vi "LaunchServerUI.vi"   [LabVIEW 2018, in "ServerUI.lvlib"]
uses:
  ServerUI.lvlib
  ServerUI/ServerUI.lvclass
  C:/Repos/AF_TCP_Example/TCP_Client/TCP_Client/TCP_Client.lvclass
  ClientUI/ClientUI/ClientUI.lvclass
  TCP_Client/TCP_Client/TCP_Client.lvclass
  C:/Program Files/National Instruments/LabVIEW 2018/vi.lib/ActorFramework/Actor/Actor.lvclass
  <vilib>/ActorFramework/Actor/Actor.lvclass
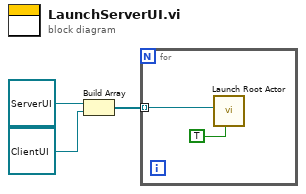
[diagram p0: block diagram]
diagram:
  n1 = Build Array(refnum<class "ServerUI.lvclass"> refnum ("ServerUI.lvlib:ServerUI.lvclass"), refnum<class "ClientUI.lvclass"> refnum ("ClientUI.lvlib:ClientUI.lvclass")) -> (w2:refnum<class "TCP_Client.lvclass">[])
  n2 = for {
    tunnel: w2 -> [w4] mode=indexing
    n3 = call <vilib>:"Launch Root Actor.vi"("Open Actor Core front panel? (F)"=TRUE, "Actor"=w4) -> ()  [unwired: 8 in, 2 out]
  }
